vi "Analog Input Voltages.vi"(8 "error in (no error)":errorcluster, 10 "Analog Input Voltages":waveform(dbl)[](array[waveform]), 11 "Baratron in":refnum<class "Baratron.lvclass">) -> (0 "error out":errorcluster, 3 "Baratron out":refnum<class "Baratron.lvclass">)   [LabVIEW 2021, in "Baratron.lvclass"]
uses:
  Baratron.lvclass
  Baratron.lvclass/Baratron.ctl
  <vilib>/ActorFramework/Actor/Actor.lvclass
  Pressure Gauges/Pressure Gauges Messages/Received Pressure Msg/Received Pressure Msg.lvclass
  <vilib>/NathanCo/Color Compare/Utilities/Colors.ctl
  C:/Program Files/National Instruments/LabVIEW 2021/vi.lib/MGI/Panel Manager/Panel Actor/Panel Actor/Panel Actor.lvclass
  C:/Program Files/National Instruments/LabVIEW 2021/vi.lib/ActorFramework/Actor/Actor.lvclass
  C:/git/Pressure-Gauges/Source/Baratron/Baratron/Baratron.lvclass
  C:/Program Files/National Instruments/LabVIEW 2021/vi.lib/NathanCo/Analog Tasks/Analog Input/Analog Input Interface Messages/Analog Input Interface Messages/Analog Input Interface Messages.lvclass
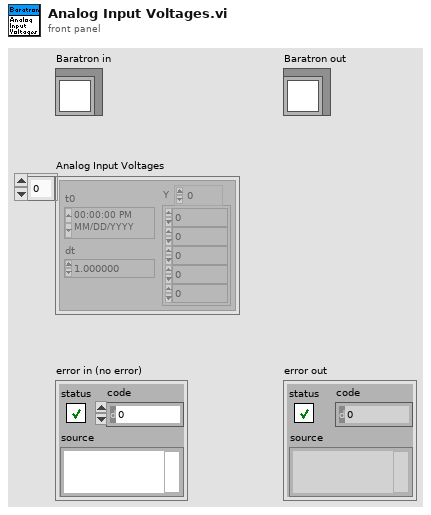
[diagram p1: front panel]
types:
  T1 = typedef "Colors.ctl" = cluster{"Green":u32, "Yellow":u32, "Red":u32}
  T2 = typedef "Baratron.lvclass/Status Range.ctl" = enum16{"Above Range", "Below Range", "Within Range"}
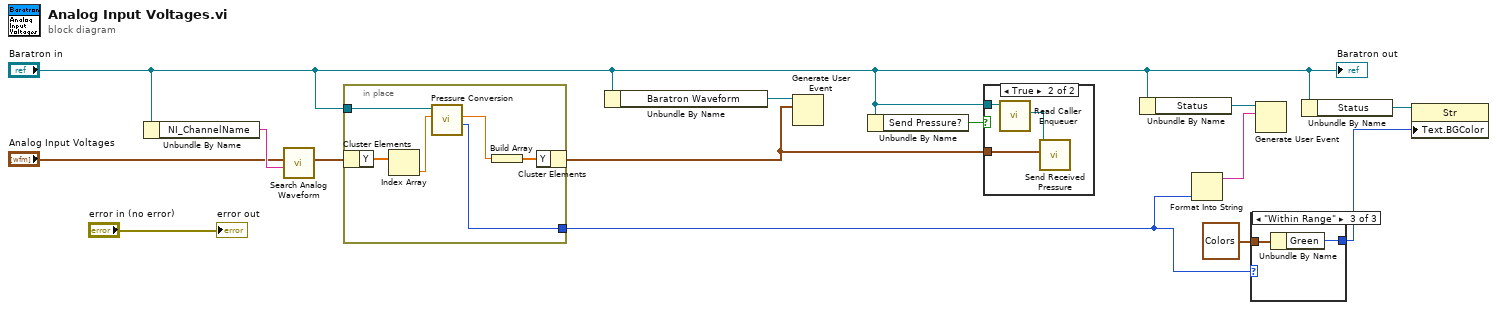
[diagram p0: block diagram]
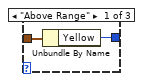
[diagram p3: hidden frame]
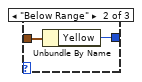
[diagram p4: hidden frame]
diagram:
  n1 = Unbundle By Name("Baratron in") -> ("NI_ChannelName"=w7:string)
  n2 = call <vilib>:"Search Analog Waveform.vi"("NI_ChannelName"=w7, "Waveforms"="Analog Input Voltages") -> ("Waveform"=w6:waveform(dbl))  [unwired: 8 in, 1 out]
  n3 = in-place {
    in-place-border: [w17] -> w1
    in-place-border: "Baratron in" -> [w16]
    n4 = in-place-cluster #1(w6) -> ("Y"=w18:dbl[])
    n5 = Index Array(array=w18) -> (element=w19:dbl)  [unwired: 1 in]
    n6 = call "Pressure Conversion.vi"("Voltage"=w19, "Baratron in"=w16) -> ("Status Range"=w17:T2, "Pressure"=w15:dbl)  [unwired: 8 in]
    n7 = Build Array(w15) -> (w20:dbl[])
    n8 = in-place-cluster #1("Y"=w20) -> (w8:waveform(dbl))
  }
  n9 = Unbundle By Name("Baratron in") -> ("Baratron Waveform"=w14:refnum<user-event>)
  n10 = Generate User Event(user event=w14, event data cluster=w8) -> ()  [unwired: 2 in, 2 out]
  n11 = Unbundle By Name("Baratron in") -> ("Send Pressure?"=w9:bool)
  n12 = case shown="True" w9 {
    tunnel: "Baratron in" -> [_ w23]
    tunnel: w8 -> [_ w21]
    frame False {
    }
    frame True {
      n13 = call <vilib>:"Read Caller Enqueuer.vi"("Actor"=w23) -> ("Caller Enqueuer"=w22:refnum<class "Message Enqueuer.lvclass">)  [unwired: 10 in]
      n14 = call "Send Received Pressure.vi"("Received Pressure"=w21, "Message Enqueuer"=w22) -> ()  [unwired: 8 in, 2 out]
    }
  }
  n15 = Unbundle By Name("Baratron in") -> ("Status"=w12:refnum<user-event>)
  n16 = Format Into String(w1) -> (resulting string=w11:string)  [unwired: 3 in, 1 out]
  n17 = case shown="\"Within Range\"" w1 {
    tunnel: [w24 w26 w28] -> w10
    tunnel: T1 {"Green"=65408, "Yellow"=16777088, "Red"=16744576} ("Colors") -> [w25 w27 w29]
    frame "Above Range" {
      n18 = Unbundle By Name(w25) -> ("Yellow"=w24:u32)
    }
    frame "Below Range" {
      n19 = Unbundle By Name(w27) -> ("Yellow"=w26:u32)
    }
    frame "Within Range" {
      n20 = Unbundle By Name(w29) -> ("Green"=w28:u32)
    }
  }
  n21 = Generate User Event(user event=w12, event data cluster=w11) -> ()  [unwired: 2 in, 2 out]
  n22 = Unbundle By Name("Baratron in") -> ("Status"=w13:refnum<vi>)
  n23 = property class="Str"(reference=w13, "Text.BGColor"=w10) -> ()  [unwired: 1 in, 2 out]
  "error out" <- "error in (no error)"
  "Baratron out" <- "Baratron in"
